vi "起始时间.vi"(9 "起始日":u16(ring), 10 "起始月":u16(ring), 11 "起始年":u16(ring)) -> (3 "起始时间":string)   [LabVIEW 2017]
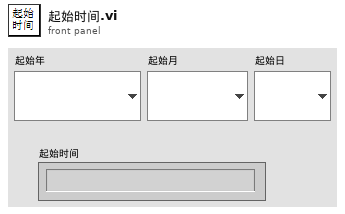
[diagram p1: front panel]
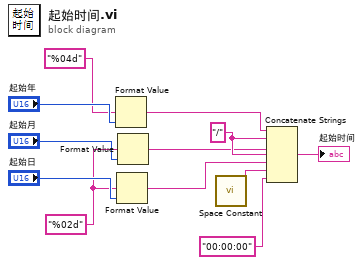
[diagram p0: block diagram]
diagram:
  w1 = "%02d" ("格式字符串")
  w11 = "/"
  n1 = Format Value(format string="%04d" ("格式字符串"), value (0)="起始年") -> (output string=w9:string)  [unwired: 1 in]
  n2 = Format Value(format string=w1, value (0)="起始日") -> (output string=w12:string)  [unwired: 1 in]
  n3 = Format Value(format string=w1, value (0)="起始月") -> (output string=w10:string)  [unwired: 1 in]
  n4 = call <vilib>:"Space Constant.vi"() -> ("String"=w8:string)
  n5 = Concatenate Strings(w9, w11, w10, w11, w12, w8, "00:00:00") -> (→"起始时间":string)
